vi "Configure Marker.vi"(5 "Marker (1)":i32=1, 7 "Channel (1)":i32=1, 8 "error in (no error)":errorcluster, 9 "Stimulus (0.0)":dbl format="%^.2e", 10 "Marker State (F: Disabled)":bool, 11 "VISA resource name":refnum<visa-resource-name>) -> (0 "error out":errorcluster, 3 "VISA resource name out":refnum<visa-resource-name>)   [LabVIEW 2018, in "Agilent ENA Series.lvlib"]
doc: "Configures marker."
uses:
  Agilent ENA Series.lvlib
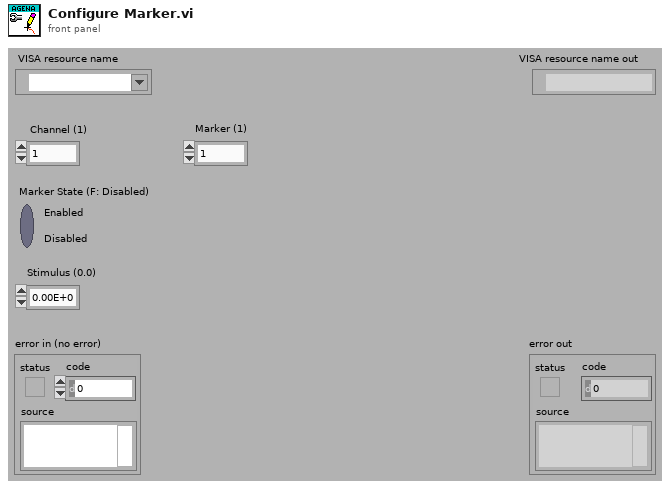
[diagram p1: front panel]
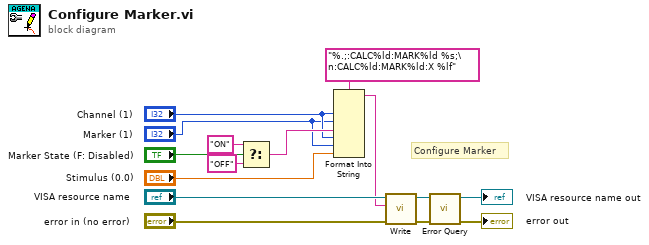
[diagram p0: block diagram]
diagram:
  # "Configure Marker"
  n1 = Select(t="ON", s="Marker State (F: Disabled)", f="OFF") -> (s? t:f=w8:string)
  n2 = Format Into String(format string="%.;:CALC%ld:MARK%ld %s;\n:CALC%ld:MARK%ld:X %lf", "Channel (1)", "Marker (1)", w8, "Channel (1)", "Marker (1)", "Stimulus (0.0)") -> (resulting string=w12:string)  [unwired: 2 in, 1 out]
  n3 = call "Write.vi"("error in (no error)"="error in (no error)", "String ()"=w12, "VISA resource name"="VISA resource name") -> ("error out"=w3:errorcluster, "VISA resource name out"=w4:refnum<visa-resource-name>)  [unwired: 6 in, 1 out]
  n4 = call "Error Query.vi"("error in (no error)"=w3, "VISA resource name"=w4) -> ("error out"=→"error out":errorcluster, "VISA resource name out"=→"VISA resource name out":refnum<visa-resource-name>)  [unwired: 6 in, 2 out]
